vi "Calc_Cross_Corr.vi"(9 "Y":dbl[](array[numeric]) format="%0.2f", 11 "X":dbl[](array[numeric]) format="%0.2f") -> (0 "Corr_Coef_Spearman":T1, 1 "Corr_Coef_Pearson":T1, 3 "Cross":dbl[](graph))   [LabVIEW 2020]
uses:
  <vilib>/Analysis/2dsp.llb/1D Cross Correlation (DBL).vi
  <vilib>/Analysis/NI_AALPro.lvlib
  <vilib>/Analysis/NI_AALBase.lvlib
  <vilib>/gmath/NI_Gmath.lvlib
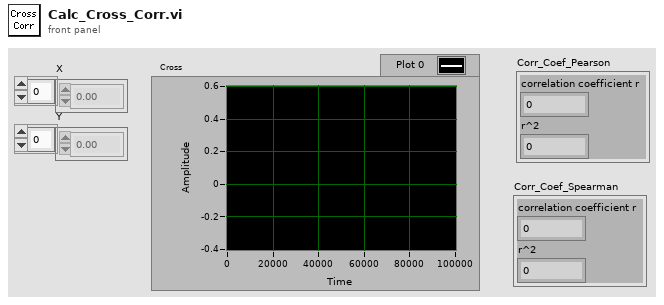
[diagram p1: front panel]
types:
  T1 = cluster{"correlation coefficient r":dbl, "r^2":dbl}
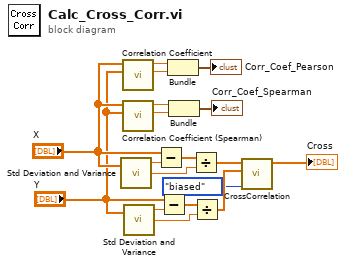
[diagram p0: block diagram]
diagram:
  n1 = call <vilib>:"Std Deviation and Variance.vi"("X"="X") -> ("mean"=w18:dbl, "standard deviation"=w16:dbl)  [unwired: 1 in, 1 out]
  n2 = call <vilib>:"Correlation Coefficient.vi"("Y"="Y", "X"="X") -> ("r^2"=w6:dbl, "correlation coefficient r"=w7:dbl)  [unwired: 8 in]
  n3 = call <vilib>:"Correlation Coefficient (Spearman).vi"("Y"="Y", "X"="X") -> ("r^2"=w2:dbl, "correlation coefficient r"=w3:dbl)  [unwired: 8 in]
  n4 = call <vilib>:"Std Deviation and Variance.vi"("X"="Y") -> ("mean"=w15:dbl, "standard deviation"=w13:dbl)  [unwired: 1 in, 1 out]
  n5 = Subtract(x="X", y=w18) -> (x-y=w17:dbl[])
  n6 = Subtract(x="Y", y=w15) -> (x-y=w14:dbl[])
  n7 = Bundle("correlation coefficient r"=w7, "r^2"=w6) -> (→"Corr_Coef_Pearson":T1)  [unwired: 1 in]
  n8 = Bundle("correlation coefficient r"=w3, "r^2"=w2) -> (→"Corr_Coef_Spearman":T1)  [unwired: 1 in]
  n9 = Divide(x=w17, y=w16) -> (x/y=w12:dbl[])
  n10 = Divide(x=w14, y=w13) -> (x/y=w11:dbl[])
  n11 = call-poly <vilib>:"CrossCorrelation.vi"("normalization"=enum32{"none", "unbiased", "biased"}."biased", "Y"=w11, "X"=w12) -> ("Rxy"=→"Cross":dbl[])  [unwired: 7 in, 1 out]
